vi "Actor Core.vi"(8 "error in":cluster{"状态":bool, "代码":i32, "源":string} caption="错误输入", 11 "仿真水位":refnum<class "Simulated Water Level.lvclass">) -> (0 "error out":cluster{"状态":bool, "代码":i32, "源":string} caption="错误输出", 3 "操作者输出":refnum<class "Actor.lvclass">)   [LabVIEW 2013, in "Simulated Water Level.lvclass"]
doc: "Actor Core.vi包含操作者的主要消息处理循环。操作者通常位于该循环中，在各种消息到达时对消息进行处理。如Do.vi消息返回任何错误，该循环将停止运行，错误代码43将被作为“无错误停止”的标准信号发送给调用方。如需更改上述行为，可在子孙类的Handle Error.vi中对该部分逻辑进行重写。"
uses:
  Simulated Water Level.lvclass
  <vilib>/ActorFramework/Actor/Actor.lvclass
  Water Level/Water Level.lvclass
  Cooler Plug-Ins/Simulated Evaporative Cooler.lvclass/Simulation Data_Global.vi
  Cooler Plug-Ins/Simulated Evaporative Cooler.lvclass/Simulated Evaporative Cooler.lvclass
panel:
  out "停止信号":bool
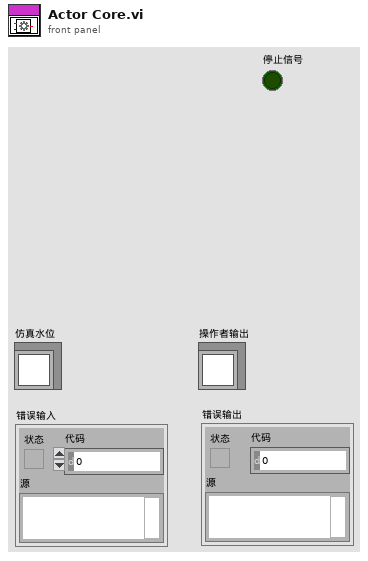
[diagram p1: front panel]
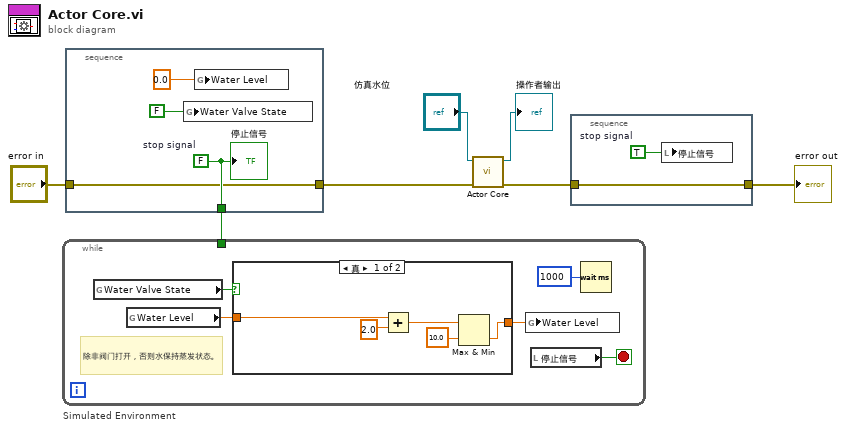
[diagram p0: block diagram]
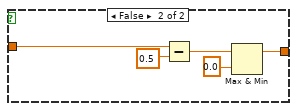
[diagram p2: hidden frame]
diagram:
  n1 = stacked-sequence {
    tunnel: [w11] -> w7
    tunnel: [w10] -> w4
    tunnel: "error in" -> [w10]
    frame #0 {
      w11 = FALSE  # stop signal
      n2 = global write "Simulation Data_Global.vi" "Water Valve State"(FALSE ("Water Valve State")) -> ()
      n3 = global write "Simulation Data_Global.vi" "Water Level"(0.0 ("Water Level")) -> ()
      "停止信号" <- w11
    }
  }
  n4 = while "Simulated Environment" {
    tunnel: w7 -> [_]
    stop <- w16 stop-if-true
    # "除非阀门打开，否则水保持蒸发状态。"
    n5 = global read "Simulation Data_Global.vi" "Water Valve State"() -> (w14:bool)
    n6 = global read "Simulation Data_Global.vi" "Water Level"() -> (w13:dbl)
    n7 = case shown="真" w14 {
      tunnel: w13 -> [w18 w23]
      tunnel: [w17 w22] -> w12
      frame True {
        n8 = Add(x=w18, y=2.0) -> (x+y=w20:dbl)
        n9 = Max & Min(x=w20, y=10.0) -> (min(x,y)=w17:dbl)  [unwired: 1 out]
      }
      frame False {
        n10 = Subtract(x=w23, y=0.5) -> (x-y=w25:dbl)
        n11 = Max & Min(x=w25, y=0.0) -> (max(x,y)=w22:dbl)  [unwired: 1 out]
      }
    }
    n12 = global write "Simulation Data_Global.vi" "Water Level"(w12) -> ()
    n13 = local read "停止信号"() -> (w16:bool)
    n14 = Wait (ms)(milliseconds to wait=u32 1000) -> ()  [unwired: 1 out]
  }
  n15 = call-parent "Actor Core.vi"("error in"=w4, "定时循环控制器"="仿真水位") -> ("error out"=w1:cluster{"状态":bool, "代码":i32, "源":string}, "操作者输出"=→"操作者输出":refnum<class "Actor.lvclass">)  [unwired: 8 in]
  n16 = stacked-sequence {
    tunnel: [w27] -> w2
    tunnel: w1 -> [w27]
    frame #0 {
      w28 = TRUE  # stop signal
      n17 = local write "停止信号"(w28) -> ()
    }
  }
  "error out" <- w2
